vi "Write GameBoard.vi"(10 "GameBoard":u8[][](array[numeric]), 11 "Analyse Board Msg in":refnum<class "Analyse Board Msg.lvclass">) -> (3 "Analyse Board Msg out":refnum<class "Analyse Board Msg.lvclass">)   [LabVIEW 2014, in "GoBang.lvlib" / "Analyse Board Msg.lvclass"]
uses:
  Analyse Board Msg.lvclass
  Analyse Board Msg.lvclass/Analyse Board Msg.ctl
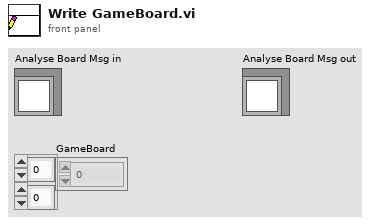
[diagram p1: front panel]
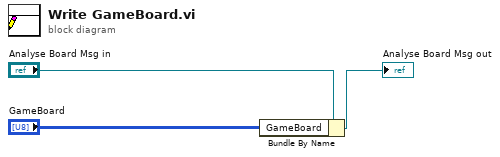
[diagram p0: block diagram]
diagram:
  n1 = Bundle By Name(cluster="Analyse Board Msg in", "GameBoard"="GameBoard") -> (→"Analyse Board Msg out":refnum<class "Analyse Board Msg.lvclass">)
